vi "Wait ms.vi"(8 "error in (no error)":errorcluster, 11 "Delay Time (ms)":dbl) -> (0 "error out":errorcluster)   [LabVIEW 2025]
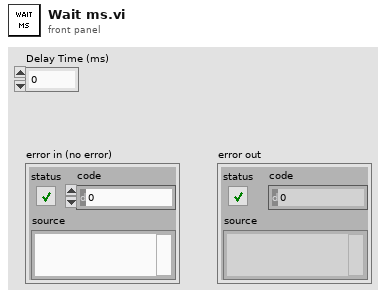
[diagram p1: front panel]
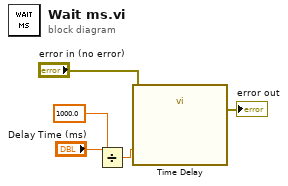
[diagram p0: block diagram]
diagram:
  n1 = Divide(x="Delay Time (ms)", y=1000.0) -> (x/y=w1:dbl)
  n2 = call "Time Delay"("error in (no error)"="error in (no error)", "Delay Time (s)"=w1) -> ("error out"=→"error out":errorcluster)  [unwired: 9 in]
